vi "Initialize.vi"(6 "optional":variant, 8 "error in":errorcluster, 11 "General in":refnum<class "General.lvclass">) -> (0 "error out":errorcluster, 3 "Node*":refnum<data-value>)   [LabVIEW 2012, in "General.lvclass"]
doc: "Initializes a xceDataNode."
uses:
  General.lvclass
  <userlib>/XCE/xCE Source/xCE/xceNode/xceNode.lvclass
  <userlib>/XCE/xCE Source/xCE/xceDataNode/xceDataNode.lvclass
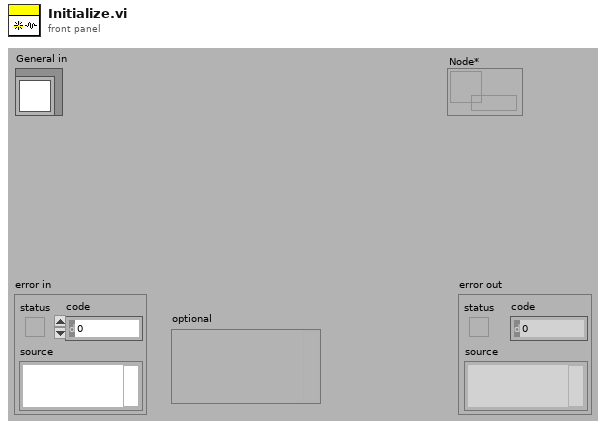
[diagram p1: front panel]
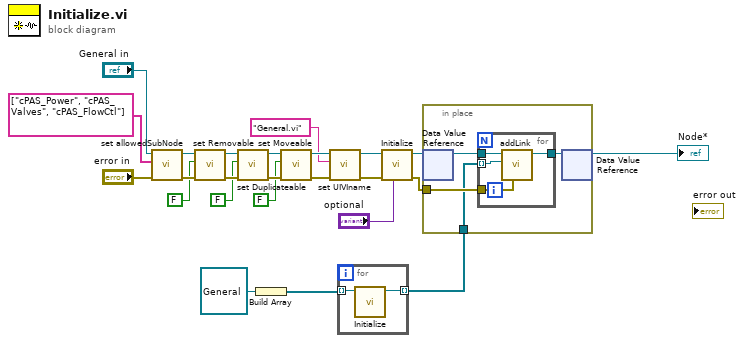
[diagram p0: block diagram]
diagram:
  n1 = call <userlib>:"set allowedSubNode.vi"("error in (no error)"="error in", "Allowed subNode[]"=string[] ["cPAS_Power", "cPAS_Valves", "cPAS_FlowCtl"], "xceDataNode in"="General in") -> ("error out"=w21:errorcluster, "xceDataNode out"=w22:refnum<class "General.lvclass">)  [unwired: 7 in]
  n2 = call <userlib>:"set Removable.vi"("error in (no error)"=w21, "Removable"=FALSE, "xceDataNode in"=w22) -> ("error out"=w19:errorcluster, "xceDataNode out"=w20:refnum<class "General.lvclass">)  [unwired: 7 in]
  n3 = call <userlib>:"set Duplicateable.vi"("error in (no error)"=w19, "Duplicateable"=FALSE, "xceDataNode in"=w20) -> ("error out"=w17:errorcluster, "xceDataNode out"=w18:refnum<class "General.lvclass">)  [unwired: 7 in]
  n4 = Build Array(refnum<class "General.lvclass"> refnum ("General.lvclass")) -> (w2:refnum<class "General.lvclass">[])
  n5 = call <userlib>:"set Moveable.vi"("error in (no error)"=w17, "Moveable"=FALSE, "xceDataNode in"=w18) -> ("error out"=w12:errorcluster, "xceDataNode out"=w13:refnum<class "General.lvclass">)  [unwired: 7 in]
  n6 = call <userlib>:"set UIVIname.vi"("error in (no error)"=w12, "UI VI name"="General.vi", "xceDataNode in"=w13) -> ("error out"=w7:errorcluster, "xceDataNode out"=w8:refnum<class "General.lvclass">)  [unwired: 7 in]
  n7 = for {
    tunnel: w2 -> [w26] mode=indexing
    tunnel: [w25] -> w1 mode=indexing
    n8 = call-dynamic "Initialize.vi"("General in"=w26) -> ("Node*"=w25:refnum<data-value>)  [unwired: 9 in, 1 out]
  }
  n9 = call-parent "Initialize.vi"("optional"="optional", "error in"=w7, "xceDataNode in"=w8) -> ("error out"=w5:errorcluster, "Node*"=w6:refnum<data-value>)  [unwired: 7 in]
  n10 = in-place {
    in-place-border: w5 -> [w29]
    in-place-border: w1 -> [w27]
    n11 = in-place-dvr #1(w6) -> (w30:refnum<class "xceNode.lvclass">)  [unwired: 1 out]
    n12 = for {
      tunnel: w30 -> [w34]
      tunnel: w29 -> [w33]
      tunnel: [w32] -> w28
      tunnel: w27 -> [w31] mode=indexing
      n13 = call <userlib>:"addLink.vi"("error in (no error)"=w33, "subNode in"=w31, "superNode in"=w34) -> ("superNode out"=w32:refnum<class "xceNode.lvclass">)  [unwired: 6 in, 2 out]
    }
    n14 = in-place-dvr #1(w28) -> (→"Node*":refnum<data-value>)  [unwired: 1 out]
  }
